vi "ParseStepInfo.vi"(8 "error in (no error)":errorcluster, 11 "Data":variant) -> (0 "error out":errorcluster, 1 "Valid?":bool, 2 "StepData":variant, 3 "StepIndex":T1)   [LabVIEW 2016, in "SeqProcessor.lvlib"]
uses:
  SeqProcessor.lvlib
  controls/StepIndex.ctl
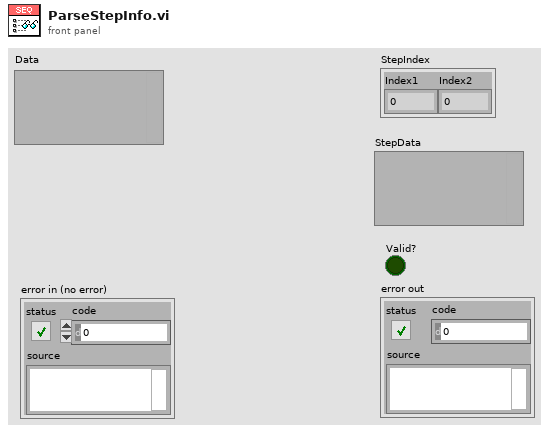
[diagram p1: front panel]
types:
  T1 = typedef "SeqProcessor.lvlib/StepIndex.ctl" = cluster{"Index1":u32, "Index2":u32}
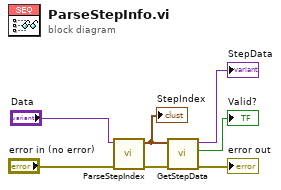
[diagram p0: block diagram]
diagram:
  n1 = call "ParseStepIndex.vi"("error in (no error)"="error in (no error)", "Data"="Data") -> ("error out"=w6:errorcluster, "StepIndex"=w7:T1)  [unwired: 8 in]
  "StepIndex" <- w7
  n2 = call "GetStepData.vi"("error in (no error)"=w6, "Index"=w7) -> ("error out"=→"error out":errorcluster, "Valid?"=→"Valid?":bool, "Data"=→"StepData":variant)  [unwired: 7 in]
